vi "Set Rx UDP.vi"(8 "error in":errorcluster, 9 "Redundant?":bool, 10 "session_tx_UDP":T2(array[cluster]), 11 "Ports Ref":T1 format="%.0x") -> (0 "error out":errorcluster, 3 "Ports Ref Out":T1 format="%.0x")   [LabVIEW 2020, in "AIM ARINC 664 Scripting.lvlib"]
uses:
  AIM ARINC 664 Scripting.lvlib
  <vilib>/NI VeriStand/Custom Device API/Custom Device Item Ref.ctl
  <vilib>/NI VeriStand/Custom Device API/Custom Device API.lvlib
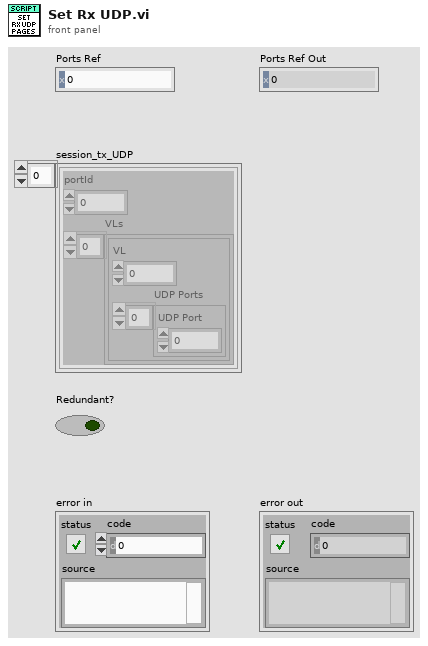
[diagram p1: front panel]
types:
  T1 = typedef "Custom Device API.lvlib/Custom Device Item Ref.ctl" = u64
  T2 = cluster{"portId":u32, "VLs":cluster{"VL":u32, "UDP Ports":u32[]}[]}[]
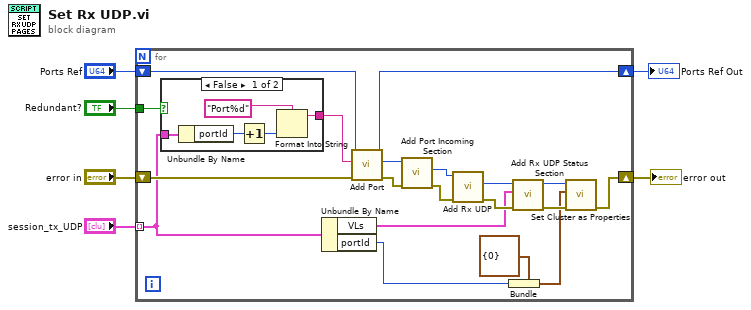
[diagram p0: block diagram]
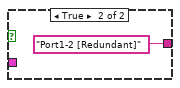
[diagram p2: hidden frame]
diagram:
  n1 = for {
    tunnel: "session_tx_UDP" -> [w13] mode=indexing
    shift-right: [w25] -> w5
    shift-left: "error in" -> [w22]
    tunnel: "Redundant?" -> [w19]
    shift-right: [w7] -> w1
    shift-left: "Ports Ref" -> [w20]
    n2 = case shown="False" w19 {
      tunnel: [w30 "Port1-2 [Redundant]"] -> w21
      tunnel: w13 -> [w27 _]
      frame False {
        n3 = Unbundle By Name(w27) -> ("portId"=w28:u32)
        n4 = Increment(x=w28) -> (x+1=w26:u32)
        n5 = Format Into String(format string="Port%d", w26) -> (resulting string=w30:string)  [unwired: 2 in, 1 out]
      }
      frame True {
      }
    }
    n6 = Unbundle By Name(w13) -> ("VLs"=w12:cluster{"VL":u32, "UDP Ports":u32[]}[], "portId"=w11:u32)
    n7 = call "Add Port.vi"("error in"=w22, "Port Name"=w21, "Ports Ref"=w20) -> ("error out"=w16:errorcluster, "Port Ref out"=w8:T1, "Parent Ref out"=w7:T1)  [unwired: 6 in]
    n8 = call "Add Port Incoming Section.vi"("error in"=w16, "Port Ref"=w8) -> ("error out"=w15:errorcluster, "Section Ptr"=w14:T1)  [unwired: 7 in, 1 out]
    n9 = call "Add Rx UDP.vi"("error in"=w15, "Port Outgoing Ref"=w14) -> ("error out"=w23:errorcluster, "Section Ptr"=w18:T1)  [unwired: 7 in, 1 out]
    n10 = Bundle(cluster=cluster{"portId":u32} {"portId"=0}, "portId"=w11) -> (w9:cluster{"portId":u32})
    n11 = call "Add Rx UDP Status Section.vi"("error in"=w23, "VLs"=w12, "Section Ref in"=w18) -> ("error out"=w24:errorcluster, "Section Ref out"=w17:T1)  [unwired: 5 in, 2 out]
    n12 = call "Set Cluster as Properties.vi"("error in"=w24, "Variant Cluster"=w9, "custom device ref in"=w17) -> ("error out"=w25:errorcluster)  [unwired: 7 in, 1 out]
  }
  "error out" <- w5
  "Ports Ref Out" <- w1
